vi "Test Modes.vi"(8 "error in (no error)":errorcluster, 11 "Instrument.Lockin in":refnum<class "Instrument.Lockin.lvclass">) -> (0 "error out":errorcluster, 3 "Instrument.Lockin out":refnum<class "Instrument.Lockin.lvclass">)   [LabVIEW 2019]
uses:
  src/Instrument.Lockin/Instrument.Lockin.lvclass
  <vilib>/addons/_JKI Toolkits/Caraya/classes/Assert/Assert Not Error.vi
  <vilib>/addons/_JKI Toolkits/Caraya/classes/Assert/Assert Not Equal Value and Type_Variant.vi
  <vilib>/addons/_JKI Toolkits/Caraya/classes/Test/Test.lvclass
  <vilib>/addons/_JKI Toolkits/Caraya/classes/Assert/Assert.lvclass
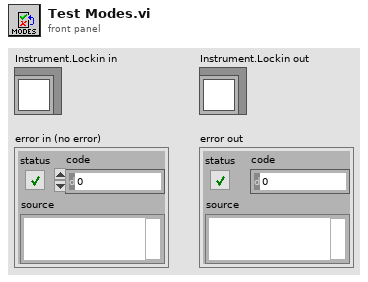
[diagram p1: front panel]
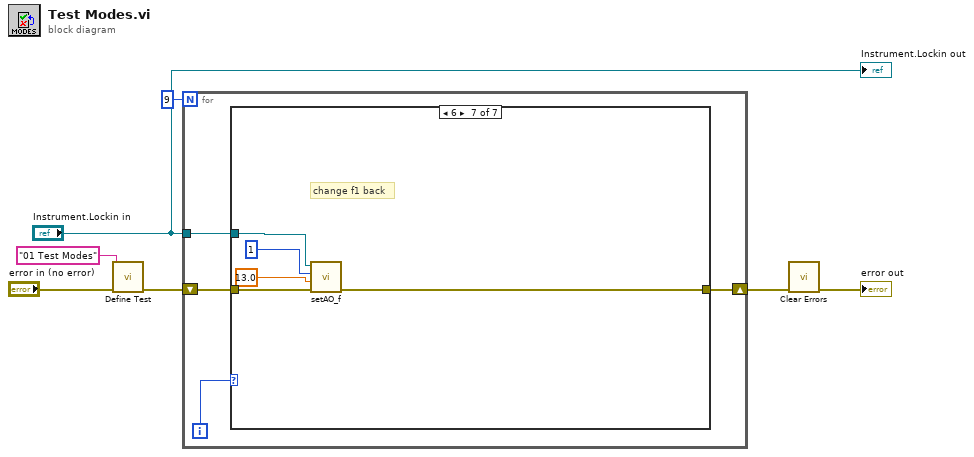
[diagram p0: block diagram]
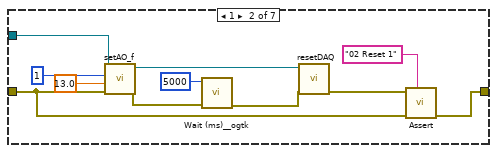
[diagram p3: hidden frame]
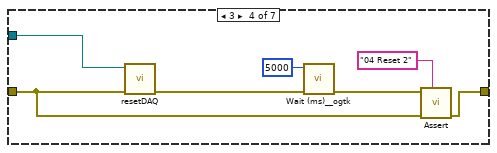
[diagram p5: hidden frame]
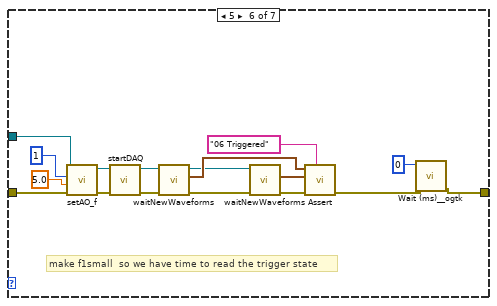
[diagram p7: hidden frame]
diagram:
  n1 = call <vilib>:"Define Test.vi"("error in (no error)"="error in (no error)", "Label (VI Title)"="01 Test Modes") -> ("error out"=w5:errorcluster)  [unwired: 8 in, 1 out]
  n2 = for {
    N: 9 -> [_]
    tunnel: "Instrument.Lockin in" -> [w8]
    shift-right: [w9] -> w4
    shift-left: w5 -> [w10]
    i -> [w11]
    n3 = case shown="6" w11 {
      tunnel: w10 -> [w12 w17 w24 w29 w32 w40 w52]
      tunnel: [w12 w13 w24 w28 w32 w35 w50] -> w9
      tunnel: w8 -> [_ w18 _ w30 _ w39 w51]
      frame 0, Default {
        # "??"
      }
      frame 1 {
        n4 = call-dynamic "setAO_f.vi"("error in (no error)"=w17, "Frequency (Hz)"=13.0, "AO Channel"=1, "Instrument.Lockin in"=w18) -> ("error out"=w15:errorcluster, "Instrument.Lockin out"=w23:refnum<class "Instrument.Lockin.lvclass">)  [unwired: 6 in]
        n5 = call <userlib>:"Wait (ms)__ogtk.vi"("error in (no error)"=w15, "milliseconds to wait"=u32 5000) -> ("error out"=w14:errorcluster)  [unwired: 8 in, 1 out]
        n6 = call-dynamic "resetDAQ.vi"("error in (no error)"=w14, "Instrument.Lockin in"=w23) -> ("error out"=w19:errorcluster)  [unwired: 8 in, 1 out]
        n7 = call-poly <vilib>:"Assert.vi"("Label"="02 Reset 1", "error in (no error)"=w17, "Not Error?"=w19) -> ("error out"=w13:errorcluster)  [unwired: 7 in, 1 out]
      }
      frame 2 {
      }
      frame 3 {
        n8 = call-dynamic "resetDAQ.vi"("error in (no error)"=w29, "Instrument.Lockin in"=w30) -> ("error out"=w26:errorcluster)  [unwired: 8 in, 1 out]
        n9 = call <userlib>:"Wait (ms)__ogtk.vi"("error in (no error)"=w26, "milliseconds to wait"=u32 5000) -> ("error out"=w25:errorcluster)  [unwired: 8 in, 1 out]
        n10 = call-poly <vilib>:"Assert.vi"("Label"="04 Reset 2", "error in (no error)"=w29, "Not Error?"=w25) -> ("error out"=w28:errorcluster)  [unwired: 7 in, 1 out]
      }
      frame 4 {
      }
      frame 5 {
        # "make f1small  so we have time to read the trigger state"
        n11 = call-dynamic "setAO_f.vi"("error in (no error)"=w40, "Frequency (Hz)"=5.0, "AO Channel"=1, "Instrument.Lockin in"=w39) -> ("error out"=w44:errorcluster, "Instrument.Lockin out"=w45:refnum<class "Instrument.Lockin.lvclass">)  [unwired: 6 in]
        n12 = call-dynamic "startDAQ.vi"("error in (no error)"=w44, "Instrument.Lockin in"=w45) -> ("error out"=w46:errorcluster, "Instrument.Lockin out"=w47:refnum<class "Instrument.Lockin.lvclass">)  [unwired: 8 in]
        n13 = call-dynamic "waitNewWaveforms.vi"("error in (no error)"=w46, "Instrument.Lockin in"=w47) -> ("error out"=w33:errorcluster, "AI Waveforms"=w38:waveform(dbl)[], "Instrument.Lockin out"=w34:refnum<class "Instrument.Lockin.lvclass">)  [unwired: 7 in]
        n14 = call-dynamic "waitNewWaveforms.vi"("error in (no error)"=w33, "Instrument.Lockin in"=w34) -> ("error out"=w49:errorcluster, "AI Waveforms"=w48:waveform(dbl)[])  [unwired: 7 in, 1 out]
        n15 = call-poly <vilib>:"Assert.vi"("Label"="06 Triggered", "error in (no error)"=w49, "Actual"=w48, "Expected"=w38) -> ("error out"=w36:errorcluster)  [unwired: 6 in, 1 out]
        n16 = call <userlib>:"Wait (ms)__ogtk.vi"("error in (no error)"=w36, "milliseconds to wait"=u32 0) -> ("error out"=w35:errorcluster)  [unwired: 8 in, 1 out]
      }
      frame 6 {
        # "change f1 back"
        n17 = call-dynamic "setAO_f.vi"("error in (no error)"=w52, "Frequency (Hz)"=13.0, "AO Channel"=1, "Instrument.Lockin in"=w51) -> ("error out"=w50:errorcluster)  [unwired: 6 in, 1 out]
      }
    }
  }
  n18 = call <vilib>:"Clear Errors.vi"("error in (no error)"=w4) -> ("error out"=→"error out":errorcluster)  [unwired: 5 in, 1 out]
  "Instrument.Lockin out" <- "Instrument.Lockin in"
